vi "Copy lvclass.vi"(6 "Name Class":string, 8 "Class Folder Path":path, 9 "Template Path":path, 10 "Application Instance":refnum<vi>) -> (0 "error out":errorcluster, 2 "New Library Path":path)   [LabVIEW 2021, in "_Template.lvlib" / "Script Strategy.lvlib"]
uses:
  Script Strategy.lvlib
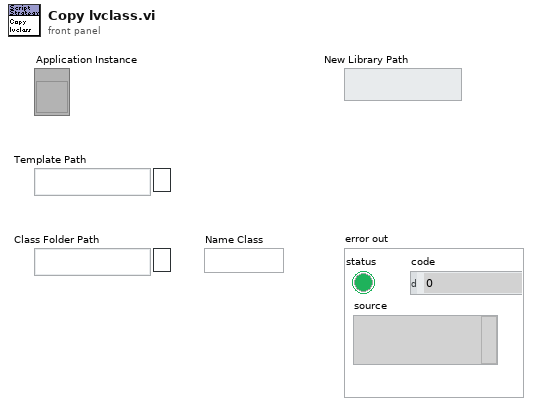
[diagram p1: front panel]
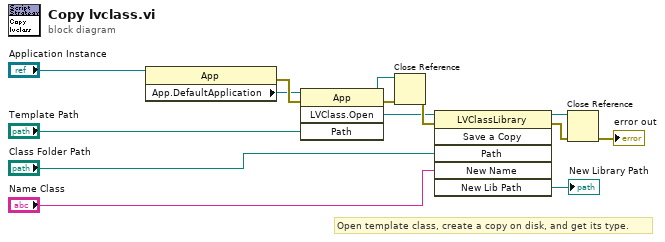
[diagram p0: block diagram]
diagram:
  # "Open template class, create a copy on disk, and get its type."
  n1 = property class="App"(reference="Application Instance") -> (error out=w13:errorcluster, "App.DefaultApplication"=w9:refnum<vi>)  [unwired: 1 in, 1 out]
  n2 = invoke class="App" method="LVClass.Open"(reference=w9, error in=w13, "Path"="Template Path") -> (reference out=w8:refnum<vi>, error out=w14:errorcluster, "LVClass.Open"=w11:refnum<vi>)  [unwired: 1 in, 1 out]
  n3 = Close Reference(reference=w8, error in (no error)=w14) -> (error out=w12:errorcluster)
  n4 = invoke class="LVClassLibrary" method="Save a Copy"(reference=w11, error in=w12, "Path"="Class Folder Path", "New Name"="Name Class") -> (reference out=w10:refnum<vi>, error out=w7:errorcluster, "New Lib Path"=→"New Library Path":path)  [unwired: 2 in, 3 out]
  n5 = Close Reference(reference=w10, error in (no error)=w7) -> (error out=→"error out":errorcluster)
